vi "Add Recipe.vi"(4 "Speed":u16, 5 "Temperature":u16, 8 "error in (no error)":errorcluster, 10 "Time Limit":u16, 11 "Masterv2 in":refnum<class "Masterv2.lvclass">) -> (0 "error out":errorcluster, 3 "Masterv2 out":refnum<class "Masterv2.lvclass">)   [LabVIEW 2014, in "Main Libraryv2.lvlib" / "Masterv2.lvclass"]
uses:
  Masterv2.lvclass
  Control/Main Libraryv2.lvlib
  Stryker/Drying Machine 06.20.2015/CONTROL/Recipes Indicators.ctl
panel:
  in  "new element/subarray":T1
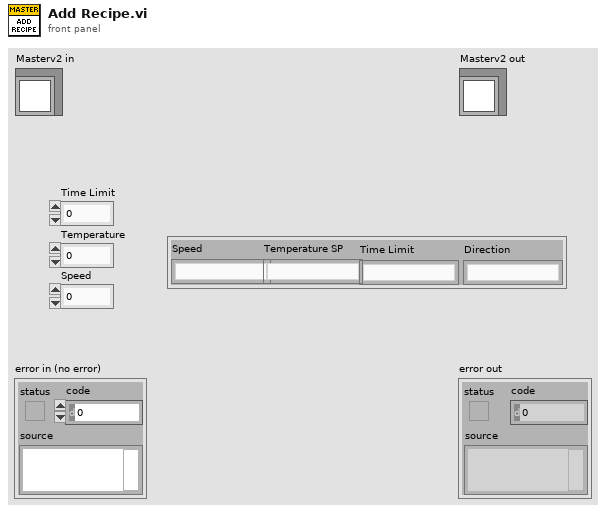
[diagram p1: front panel]
types:
  T1 = typedef "Files Library.lvlib/CONTROL LIBRARY.lvlib/Recipes Indicators.ctl" = cluster{"Speed":string, "Temperature SP":string, "Time Limit":string, "Direction":string}
  T2 = cluster{"Speed":string, "Temperature SP":string, "Time Limit":string, "Direction":string}[]
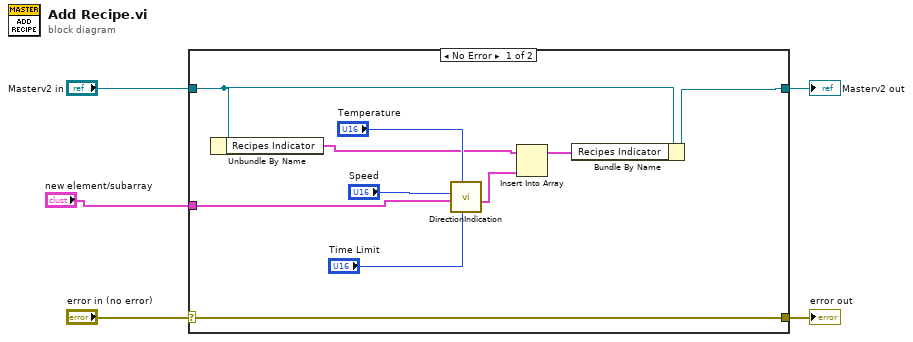
[diagram p0: block diagram]
diagram:
  n1 = case shown="No Error" "error in (no error)" {
    selector: "error in (no error)" -> [w15 w17]
    tunnel: [w15 w17] -> w4
    tunnel: [w6 w16] -> w2
    tunnel: "Masterv2 in" -> [w7 w16]
    tunnel: "new element/subarray" -> [w11 _]
    frame No Error {
      n2 = Unbundle By Name(w7) -> ("Recipes Indicator"=w10:T2)
      n3 = call "DirectionIndication.vi"("Time Limit"="Time Limit", "Temperature"="Temperature", "new element/subarray 2"=w11, "Speed"="Speed") -> ("new element/subarray 3"=w9:T1)  [unwired: 7 in]
      n4 = Insert Into Array(array=w10, new element=w9) -> (w8:T2)  [unwired: 1 in]
      n5 = Bundle By Name(cluster=w7, "Recipes Indicator"=w8) -> (w6:refnum<class "Masterv2.lvclass">)
    }
    frame Error {
    }
  }
  "error out" <- w4
  "Masterv2 out" <- w2
